vi "32-bit Counter.vi"(8 "INC?":bool, 10 "Reset?":bool, 11 "rollover":u32) -> (3 "count":u32)   [LabVIEW 2012]
doc: "This counter counts from 0....Rollover and then returns to zero\ne.g., If rollover is 2, counter moves as 0,1,2,0,1,2.....\n\n<Latency> = 1 Tick from Reset"
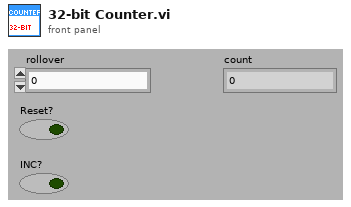
[diagram p1: front panel]
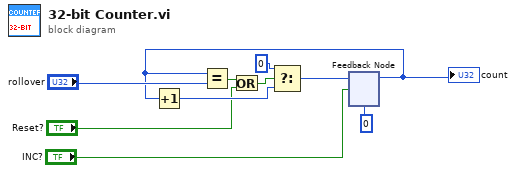
[diagram p0: block diagram]
diagram:
  n1 = feedback #1(u32 0) -> (w1:u32)
  "count" <- w1
  n2 = Increment(x=w1) -> (x+1=w5:u32)
  n3 = Equal?(x=w1, y="rollover") -> (x = y?=w8:bool)
  n4 = Or(x=w8, y="Reset?") -> (x .or. y?=w7:bool)
  n5 = Select(t=u32 0, s=w7, f=w5) -> (s? t:f=w6:u32)
  n6 = feedback-in #1(w6, "INC?") -> ()
